vi "PLC Primitive Byte Stream to G Object.vi"(8 "error in (no error)":errorcluster, 9 "PLC Type":T1, 10 "Byte Stream":u8[](array[numeric]), 11 "TwinCAT ADS in":refnum<class "TwinCAT ADS.lvclass">) -> (0 "error out":errorcluster, 2 "Value":variant, 3 "TwinCAT ADS out":refnum<class "TwinCAT ADS.lvclass">)   [LabVIEW 2018, in "TwinCAT ADS.lvclass"]
uses:
  TwinCAT ADS.lvclass
  Controls/PLC Type.ctl
  dd5e40b3-f89d-44d0-b911-1f2dc1f1e391.vi
  9a8c356b-cf55-4838-9201-0532b80217b2.vi
  06482052-d1f9-4f29-aca9-908031c6a69f.vi
  b9242781-96b0-446e-9150-452b1084ed54.vi
  5fbe6976-0b86-40a2-b7b6-3748894f0071.vi
  c4de1741-fffd-4fed-ba25-d7b4acbf0555.vi
  20356124-05d2-4a04-a5d1-e69adc4c58c2.vi
  67ddb754-0fbe-43d9-9e61-34d6659124ef.vi
  e3d41cb3-d20e-45e9-8252-e41884a8f4d0.vi
  46ba2a54-cc07-4222-9a0e-bd972edfcef0.vi
  6b416cf7-30dc-48a3-9278-9d800f443678.vi
  5857d013-9824-4299-a2d7-53efdc0d26c5.vi
  006b0e7e-7e80-41f3-be4e-1f3da8479fae.vi
  28d9c90b-5f2a-4c58-95e2-5fc46303b0fd.vi
  99b7bc4a-962e-4818-aa5d-444f23f83b11.vi
  8b7c42c8-9170-4542-8f35-15cbeddc22cb.vi
  65a091fa-0bd2-4a35-ae2b-3fa5e90d1994.vi
  4b7d3a7d-7f1b-46f0-9357-48cb72148c56.vi
  b431183c-2ad5-4c6d-9bfa-a53b18913682.vi
  30c6c28a-53c3-4e33-80b1-b22f521e1f67.vi
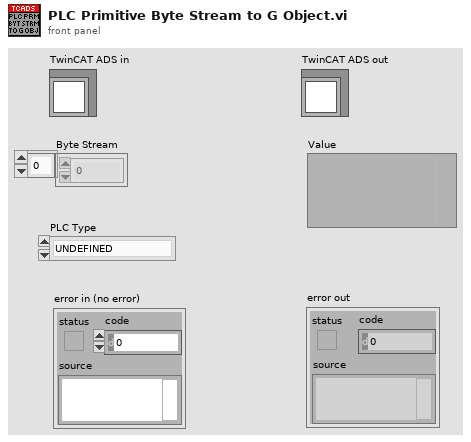
[diagram p1: front panel]
types:
  T1 = typedef "TwinCAT ADS.lvclass/PLC Type.ctl" = enum16{"UNDEFINED", "INT", "DINT", "REAL", "LREAL", "SINT", "BYTE", "UINT", "UDINT", "LINT", "ULINT", "STRING", "WSTRING", "BOOL", "TIME", "LTIME", "DATE", "DT", "TOD", "ARRAY", "JAGGED ARRAY", "STRUCT", "FUNCTION BLOCK", "UNION", "POINTER", "USER DEFINED"}
  T2 = typedef "LVDateTimeRec.ctl" = cluster{"fractional second":dbl, "second":i32, "minute":i32, "hour":i32, "day of month":i32, "month":i32, "year":i32, "day of week":i32, "day of year":i32, "DST":i32}
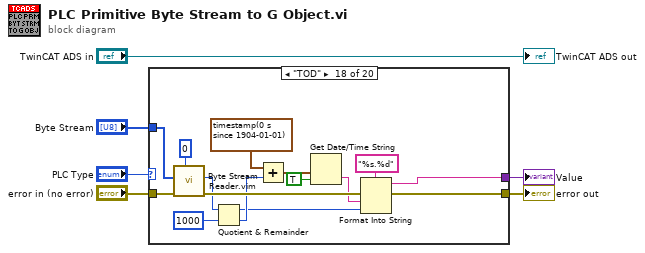
[diagram p0: block diagram]
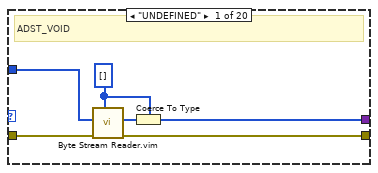
[diagram p2: hidden frame]
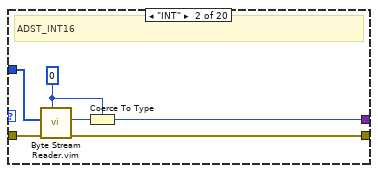
[diagram p3: hidden frame]
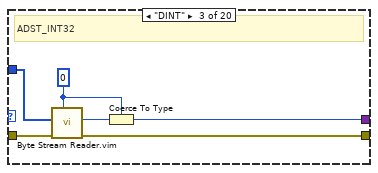
[diagram p4: hidden frame]
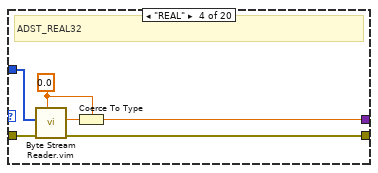
[diagram p5: hidden frame]
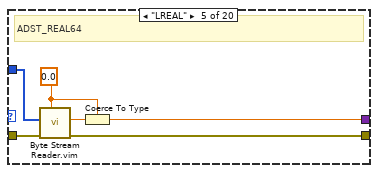
[diagram p6: hidden frame]
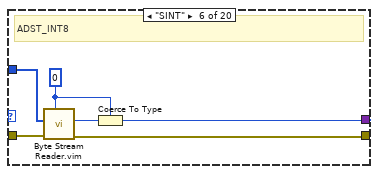
[diagram p7: hidden frame]
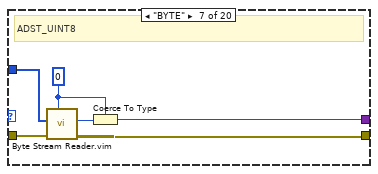
[diagram p8: hidden frame]
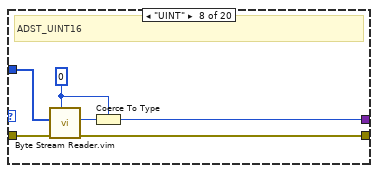
[diagram p9: hidden frame]
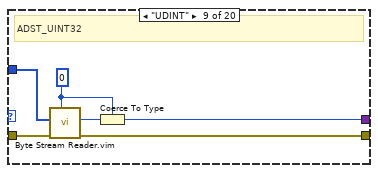
[diagram p10: hidden frame]
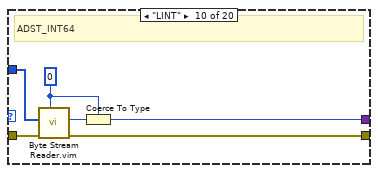
[diagram p11: hidden frame]
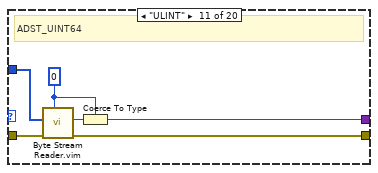
[diagram p12: hidden frame]
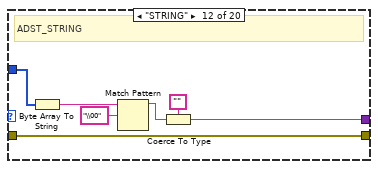
[diagram p13: hidden frame]
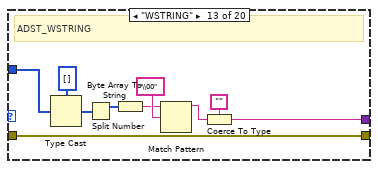
[diagram p14: hidden frame]
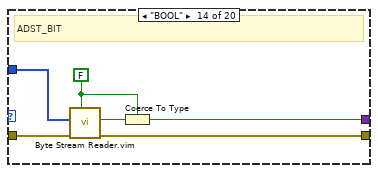
[diagram p15: hidden frame]
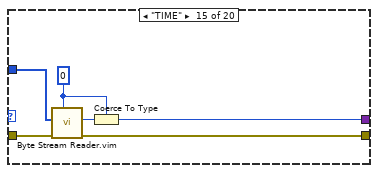
[diagram p16: hidden frame]
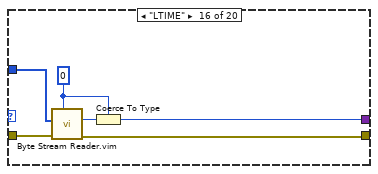
[diagram p17: hidden frame]
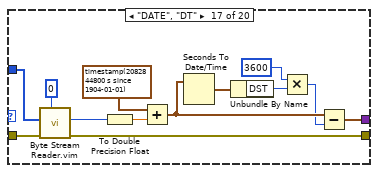
[diagram p18: hidden frame]
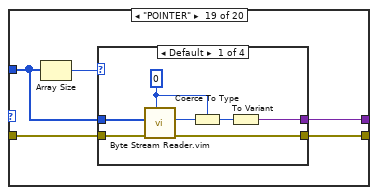
[diagram p19: hidden frame]
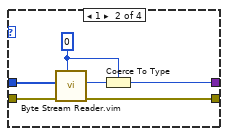
[diagram p20: hidden frame]
diagram:
  n1 = case shown="\"TOD\"" "PLC Type" {
    tunnel: [w8 w13 w19 w25 w31 w37 w43 w49 w55 w61 w67 w73 w80 w90 w97 w102 w108 w126 w137 w166] -> w4
    tunnel: "error in (no error)" -> [w11 w18 w24 w30 w36 w42 w48 w54 w60 w66 w72 w76 w83 w95 w101 w107 w119 w134 w140 w167]
    tunnel: [w7 w17 w23 w29 w35 w41 w47 w53 w58 w64 w70 w76 w83 w93 w99 w105 w116 w124 w136 w167] -> w3
    tunnel: "Byte Stream" -> [w10 w16 w22 w28 w34 w40 w46 w52 w59 w65 w71 w79 w88 w94 w100 w106 w118 w132 w138 w166]
    frame "UNDEFINED" {
      w9 = u8[] []
      # "ADST_VOID"
      n2 = call "Byte Stream Reader.vim"("Type"=w9, "error in (no error)"=w11, "Byte Stream"=w10) -> ("error out"=w7:errorcluster, "Value"=w12:u8[])  [unwired: 7 in]
      n3 = Coerce To Type(0:w12, 1:w9) -> (2:w8:u8[])
    }
    frame "INT" {
      w14 = i16 0
      # "ADST_INT16"
      n4 = call "Byte Stream Reader.vim"("Type"=w14, "error in (no error)"=w18, "Byte Stream"=w16) -> ("error out"=w17:errorcluster, "Value"=w15:i16)  [unwired: 7 in]
      n5 = Coerce To Type(0:w15, 1:w14) -> (2:w13:i16)
    }
    frame "DINT" {
      w20 = 0
      # "ADST_INT32"
      n6 = call "Byte Stream Reader.vim"("Type"=w20, "error in (no error)"=w24, "Byte Stream"=w22) -> ("error out"=w23:errorcluster, "Value"=w21:i32)  [unwired: 7 in]
      n7 = Coerce To Type(0:w21, 1:w20) -> (2:w19:i32)
    }
    frame "REAL" {
      w26 = sgl 0.0
      # "ADST_REAL32"
      n8 = call "Byte Stream Reader.vim"("Type"=w26, "error in (no error)"=w30, "Byte Stream"=w28) -> ("error out"=w29:errorcluster, "Value"=w27:sgl)  [unwired: 7 in]
      n9 = Coerce To Type(0:w27, 1:w26) -> (2:w25:sgl)
    }
    frame "LREAL" {
      w32 = 0.0
      # "ADST_REAL64"
      n10 = call "Byte Stream Reader.vim"("Type"=w32, "error in (no error)"=w36, "Byte Stream"=w34) -> ("error out"=w35:errorcluster, "Value"=w33:dbl)  [unwired: 7 in]
      n11 = Coerce To Type(0:w33, 1:w32) -> (2:w31:dbl)
    }
    frame "SINT" {
      w38 = i8 0
      # "ADST_INT8"
      n12 = call "Byte Stream Reader.vim"("Type"=w38, "error in (no error)"=w42, "Byte Stream"=w40) -> ("error out"=w41:errorcluster, "Value"=w39:i8)  [unwired: 7 in]
      n13 = Coerce To Type(0:w39, 1:w38) -> (2:w37:i8)
    }
    frame "BYTE" {
      w44 = u8 0
      # "ADST_UINT8"
      n14 = call "Byte Stream Reader.vim"("Type"=w44, "error in (no error)"=w48, "Byte Stream"=w46) -> ("error out"=w47:errorcluster, "Value"=w45:u8)  [unwired: 7 in]
      n15 = Coerce To Type(0:w45, 1:w44) -> (2:w43:u8)
    }
    frame "UINT" {
      w50 = u16 0
      # "ADST_UINT16"
      n16 = call "Byte Stream Reader.vim"("Type"=w50, "error in (no error)"=w54, "Byte Stream"=w52) -> ("error out"=w53:errorcluster, "Value"=w51:u16)  [unwired: 7 in]
      n17 = Coerce To Type(0:w51, 1:w50) -> (2:w49:u16)
    }
    frame "UDINT" {
      w56 = u32 0
      # "ADST_UINT32"
      n18 = call "Byte Stream Reader.vim"("Type"=w56, "error in (no error)"=w60, "Byte Stream"=w59) -> ("error out"=w58:errorcluster, "Value"=w57:u32)  [unwired: 7 in]
      n19 = Coerce To Type(0:w57, 1:w56) -> (2:w55:u32)
    }
    frame "LINT" {
      w62 = i64 0
      # "ADST_INT64"
      n20 = call "Byte Stream Reader.vim"("Type"=w62, "error in (no error)"=w66, "Byte Stream"=w65) -> ("error out"=w64:errorcluster, "Value"=w63:i64)  [unwired: 7 in]
      n21 = Coerce To Type(0:w63, 1:w62) -> (2:w61:i64)
    }
    frame "ULINT" {
      w69 = u64 0
      # "ADST_UINT64"
      n22 = call "Byte Stream Reader.vim"("Type"=w69, "error in (no error)"=w72, "Byte Stream"=w71) -> ("error out"=w70:errorcluster, "Value"=w68:u64)  [unwired: 7 in]
      n23 = Coerce To Type(0:w68, 1:w69) -> (2:w67:u64)
    }
    frame "STRING" {
      # "ADST_STRING"
      n24 = Byte Array To String(unsigned byte array=w79) -> (string=w78:string)
      n25 = Match Pattern(string=w78, regular expression="\\00") -> (before substring=w74:string)  [unwired: 1 in, 3 out]
      n26 = Coerce To Type(0:w74, 1:"") -> (2:w73:string)
    }
    frame "WSTRING" {
      # "ADST_WSTRING"
      n27 = Type Cast(type=u16[] [] ("Byte Stream"), x=w88) -> (*(type *) &x=w84:u16[])
      n28 = Split Number(x=w84) -> (hi(x)=w85:u8[])  [unwired: 1 out]
      n29 = Byte Array To String(unsigned byte array=w85) -> (string=w86:string)
      n30 = Match Pattern(string=w86, regular expression="\\00") -> (before substring=w81:string)  [unwired: 1 in, 3 out]
      n31 = Coerce To Type(0:w81, 1:"") -> (2:w80:string)
    }
    frame "BOOL" {
      w91 = FALSE
      # "ADST_BIT"
      n32 = call "Byte Stream Reader.vim"("Type"=w91, "error in (no error)"=w95, "Byte Stream"=w94) -> ("error out"=w93:errorcluster, "Value"=w92:bool)  [unwired: 7 in]
      n33 = Coerce To Type(0:w92, 1:w91) -> (2:w90:bool)
    }
    frame "TIME" {
      w96 = u32 0
      n34 = call "Byte Stream Reader.vim"("Type"=w96, "error in (no error)"=w101, "Byte Stream"=w100) -> ("error out"=w99:errorcluster, "Value"=w98:u32)  [unwired: 7 in]
      n35 = Coerce To Type(0:w98, 1:w96) -> (2:w97:u32)
    }
    frame "LTIME" {
      w103 = u64 0
      n36 = call "Byte Stream Reader.vim"("Type"=w103, "error in (no error)"=w107, "Byte Stream"=w106) -> ("error out"=w105:errorcluster, "Value"=w104:u64)  [unwired: 7 in]
      n37 = Coerce To Type(0:w104, 1:w103) -> (2:w102:u64)
    }
    frame "DATE", "DT" {
      n38 = call "Byte Stream Reader.vim"("Type"=u32 0, "error in (no error)"=w119, "Byte Stream"=w118) -> ("error out"=w116:errorcluster, "Value"=w115:u32)  [unwired: 7 in]
      n39 = To Double Precision Float(number=w115) -> (double precision float=w117:dbl)
      n40 = Add(x=timestamp(2082844800 s since 1904-01-01) ("time stamp"), y=w117) -> (x+y=w113:timestamp)
      n41 = Seconds To Date/Time(time stamp (now)=w113) -> (date time rec=w112:T2)  [unwired: 1 in]
      n42 = Unbundle By Name(w112) -> ("DST"=w111:i32)
      n43 = Multiply(x=3600, y=w111) -> (x*y=w109:i32)
      n44 = Subtract(x=w113, y=w109) -> (x-y=w108:timestamp)
    }
    frame "TOD" {
      n45 = call "Byte Stream Reader.vim"("Type"=u32 0, "error in (no error)"=w134, "Byte Stream"=w132) -> ("error out"=w135:errorcluster, "Value"=w123:u32)  [unwired: 7 in]
      n46 = Quotient & Remainder(x=w123, y=u32 1000) -> (x-y*floor(x/y)=w122:u32, floor(x/y)=w129:u32)
      n47 = Add(x=timestamp(0 s since 1904-01-01), y=w129) -> (x+y=w128:timestamp)
      n48 = Get Date/Time String(seconds (now)=w128, want seconds? (F)=TRUE) -> (time string=w121:string)  [unwired: 1 in, 1 out]
      n49 = Format Into String(format string="%s.%d", error in=w135, w121, w122) -> (resulting string=w126:string, error out=w124:errorcluster)  [unwired: 1 in]
    }
    frame "POINTER" {
      n50 = Array Size(array=w138) -> (size(s)=w139:i32)
      n51 = case shown="Default" w139 {
        tunnel: w140 -> [w146 w152 w158 w164]
        tunnel: w138 -> [w144 w150 w156 w162]
        tunnel: [w143 w149 w155 w161] -> w136
        tunnel: [w141 w148 w154 w160] -> w137
        frame Default {
          w145 = u64 0
          n52 = call "Byte Stream Reader.vim"("Type"=w145, "error in (no error)"=w146, "Byte Stream"=w144) -> ("error out"=w143:errorcluster, "Value"=w147:u64)  [unwired: 7 in]
          n53 = Coerce To Type(0:w147, 1:w145) -> (2:w142:u64)
          n54 = To Variant(anything=w142) -> (Variant=w141:variant)
        }
        frame 1 {
          w151 = u64 0
          n55 = call "Byte Stream Reader.vim"("Type"=w151, "error in (no error)"=w152, "Byte Stream"=w150) -> ("error out"=w149:errorcluster, "Value"=w153:u64)  [unwired: 7 in]
          n56 = Coerce To Type(0:w153, 1:w151) -> (2:w148:u64)
        }
        frame 2 {
          w157 = u16 0
          n57 = call "Byte Stream Reader.vim"("Type"=w157, "error in (no error)"=w158, "Byte Stream"=w156) -> ("error out"=w155:errorcluster, "Value"=w159:u16)  [unwired: 7 in]
          n58 = Coerce To Type(0:w159, 1:w157) -> (2:w154:u16)
        }
        frame 4 {
          w163 = u32 0
          n59 = call "Byte Stream Reader.vim"("Type"=w163, "error in (no error)"=w164, "Byte Stream"=w162) -> ("error out"=w161:errorcluster, "Value"=w165:u32)  [unwired: 7 in]
          n60 = Coerce To Type(0:w165, 1:w163) -> (2:w160:u32)
        }
      }
    }
    frame Default {
    }
  }
  "error out" <- w3
  "Value" <- w4
  "TwinCAT ADS out" <- "TwinCAT ADS in"
